vi "important.vi"   [LabVIEW 2014]
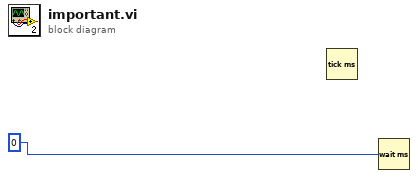
[diagram p0: block diagram]
diagram:
  n1 = Tick Count (ms)() -> ()  [unwired: 1 out]
  n2 = Wait (ms)(milliseconds to wait=0) -> ()  [unwired: 1 out]
